vi "CloseMovieFile.vi"(2 "error out":errorcluster, 3 "QT Ref Out":T1) -> ()   [LabVIEW 2024]
doc: "This VI does the necessary memory clean-up work at the end of an OpenMovieFile based vi. It is important to use this vi to prevent memory leaks and crashes."
uses:
  <userlib>/ImageProcessing/QTLIB_2595_LV86/QT_Private.ctl
  <userlib>/ImageProcessing/QTLIB_2595_LV86/QT_Ref.ctl
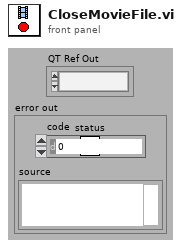
[diagram p1: front panel]
types:
  T1 = typedef "QT_Ref.ctl" = refnum<k1>
  T2 = typedef "QT_Private.ctl" = cluster{"reserved 1":i32, "reserved 2":i32, "reserved 3":i32, "reserved 4":i32}
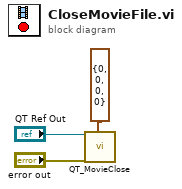
[diagram p0: block diagram]
diagram:
  n1 = call <userlib>:"QT_MovieClose.vi"("QT Ref In"="QT Ref Out", "error in (no error)"="error out", "Private"=T2 {"reserved 1"=0, "reserved 2"=0, "reserved 3"=0, "reserved 4"=0}) -> ()  [unwired: 15 in, 2 out]
